vi "AFT Filter Signal and Update Coefficients (Complex, PtByPt).vi"(6 "step size":dbl=-1.0, 7 "reset? (F)":bool, 8 "error in (no error)":errorcluster, 9 "d(n)":cdb, 10 "x(n)":cdb, 11 "adaptive filter in":refnum<k20>) -> (0 "error out":errorcluster, 1 "e(n)":cdb, 2 "y(n)":cdb, 3 "adaptive filter out":refnum<k20>)   [LabVIEW 2017, in "NI_AdaptiveFilter.lvlib"]
doc: "Filters an input signal with an adaptive filter and updates the coefficients of the adaptive filter iteratively. You must use the least mean squares (LMS) or recursive least squares (RLS) algorithms to create the adaptive filter. Wire data to the <B>x(n)</B> and <B>d(n)</B> inputs to determine the polymorphic instance to use or manually select the instance. The data type of the adaptive filter that you wire to the <B>adaptive filter in</B> input must match the instance of the AFT Filter Signal and Update Coefficients VI."
uses:
  <vilib>/addons/Adaptive Filters/NI_AdaptiveFilter.lvlib
  <resource>/AdaptiveFilters.dll
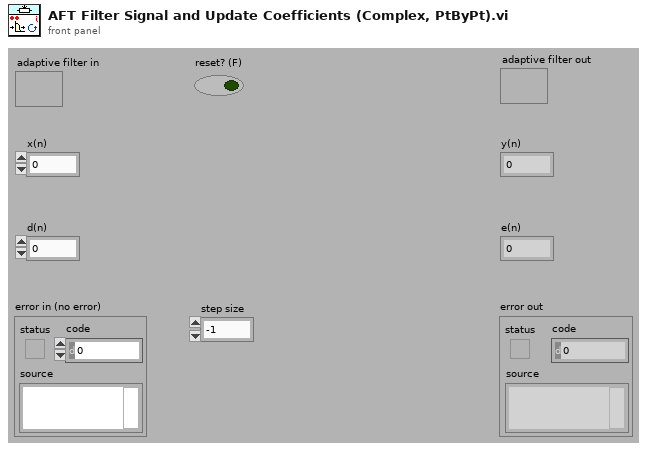
[diagram p1: front panel]
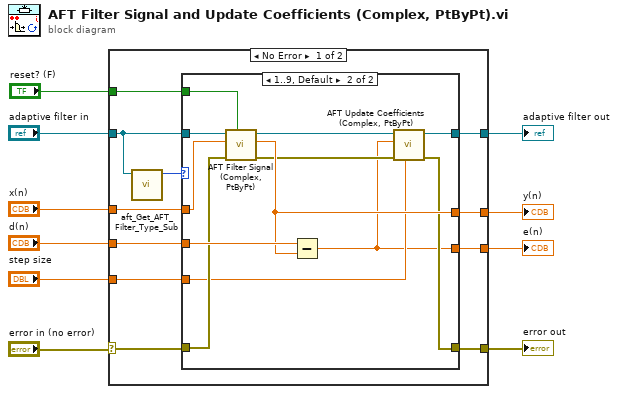
[diagram p0: block diagram]
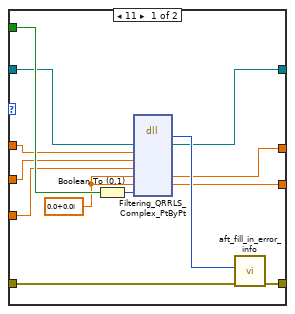
[diagram p2: hidden frame]
diagram:
  n1 = case shown="No Error" "error in (no error)" {
    selector: "error in (no error)" -> [w18 w48]
    tunnel: [w17 w48] -> w10
    tunnel: "adaptive filter in" -> [w13 w47]
    tunnel: "x(n)" -> [w21 _]
    tunnel: "d(n)" -> [w20 _]
    tunnel: [w12 w47] -> w5
    tunnel: "step size" -> [w16 _]
    tunnel: [w19 _] -> w3
    tunnel: [w14 _] -> w2
    tunnel: "reset? (F)" -> [w15 _]
    frame No Error {
      n2 = call <vilib>:"aft_Get_AFT_Filter_Type_Sub.vi"("adaptive filter in"=w13) -> ("type"=w11:i32)  [unwired: 9 out]
      n3 = case shown="1..9, Default" w11 {
        tunnel: w21 -> [w24 w46]
        tunnel: w20 -> [w29 w45]
        tunnel: [w26 w44] -> w19
        tunnel: w13 -> [w23 w42]
        tunnel: w18 -> [w32 w41]
        tunnel: [w31 w40] -> w17
        tunnel: w16 -> [w27 w38]
        tunnel: w15 -> [w30 w37]
        tunnel: [w25 w35] -> w14
        tunnel: [w22 w36] -> w12
        frame 11 {
          w28 = cdb 0.0+0.0i ("x(n)")
          n4 = Boolean To (0,1)(Boolean=w30) -> (0, 1=w34:i16)
          n5 = dll-call lib="C:/Program Files/National Instruments/LabVIEW 2017/resource/AdaptiveFilters.dll" fn="Filtering_QRRLS_Complex_PtByPt" ("Complex Data Initialization")("pSession"=w23, "x"=w24, "d"=w29, "mu"=w27, "y"=w28, "e"=w28, "reset"=w34) -> ("err"=w33:i32, "pSession"=w22:refnum<k20>, "y"=w26:cdb, "e"=w25:cdb)  [unwired: 7 in, 2 out]
          n6 = call <vilib>:"aft_fill_in_error_info.vi"("error in"=w32, "status code"=w33) -> ("error out"=w31:errorcluster)  [unwired: 2 in, 7 out]
        }
        frame 1..9, Default {
          n7 = call <vilib>:"AFT Filter Signal (Complex, PtByPt).vi"("reset? (F)"=w37, "error in (no error)"=w41, "x(n)"=w46, "adaptive filter in"=w42) -> ("error out"=w39:errorcluster, "y(n)"=w44:cdb, "adaptive filter out"=w43:refnum<k20>)  [unwired: 5 out]
          n8 = Subtract(x=w45, y=w44) -> (x-y=w35:cdb)
          n9 = call <vilib>:"AFT Update Coefficients (Complex, PtByPt).vi"("step size"=w38, "error in (no error)"=w39, "e(n)"=w35, "adaptive filter in"=w43) -> ("error out"=w40:errorcluster, "adaptive filter out"=w36:refnum<k20>)  [unwired: 6 out]
        }
      }
    }
    frame Error {
    }
  }
  "error out" <- w10
  "y(n)" <- w3
  "e(n)" <- w2
  "adaptive filter out" <- w5
